vi "ID_ja_aberto.vi"(8 "Conexao nova":refnum<k5>, 9 "Conexao fechada":refnum<k5>, 11 "Entrada Array Conexao":refnum<k5>[](array[refnum])) -> (0 "Saida Array Conexao":refnum<k5>[](array[refnum]))   [LabVIEW 2019]
panel:
  out "iguais":dbl
  # "VI responsável para fazer o controle se o ID recebido é um ID já aberto ou não, e caso ele for fechado, não adicioná-lo"
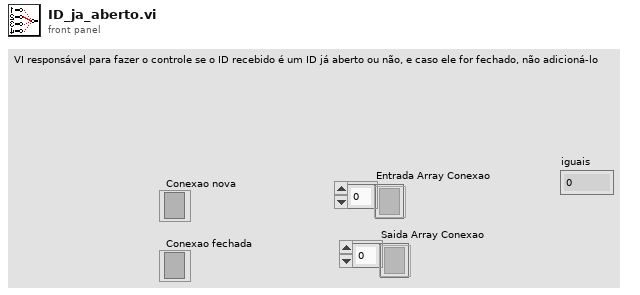
[diagram p1: front panel]
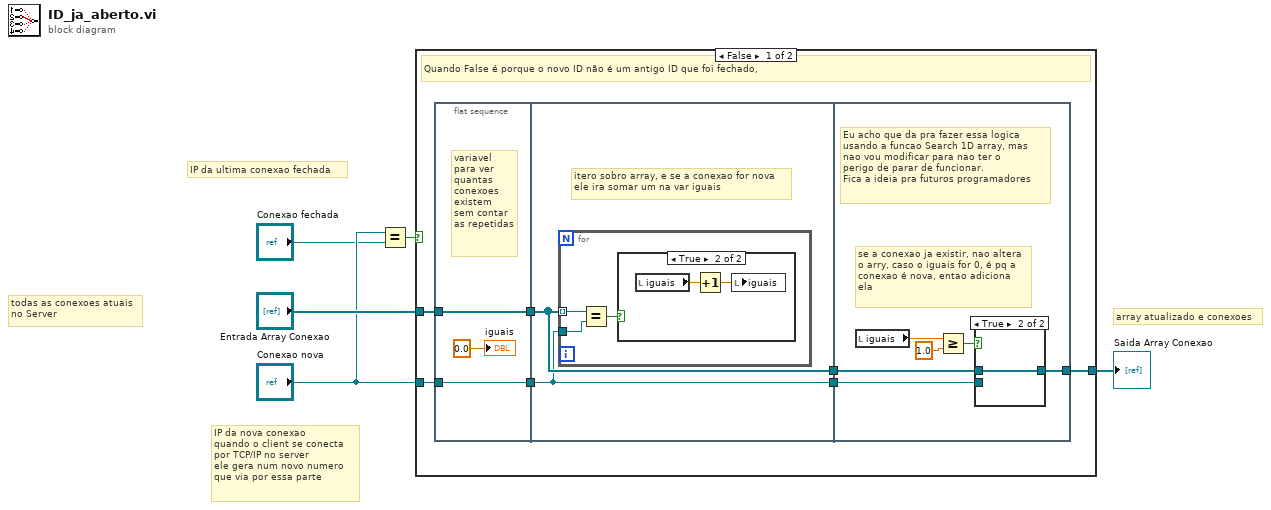
[diagram p0: block diagram]
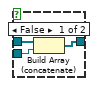
[diagram p3: hidden frame]
diagram:
  # "array atualizado e conexoes"
  # "todas as conexoes atuais\nno Server"
  # "IP da nova conexao\nquando o client se conecta\npor TCP/IP no server\nele gera num novo numero\nque via por essa parte"
  # "IP da ultima conexao fechada"
  n1 = Equal?(x="Conexao nova", y="Conexao fechada") -> (x = y?=w1:bool)
  n2 = case shown="False" w1 {
    tunnel: [w10 w33] -> w5
    tunnel: "Entrada Array Conexao" -> [w8 w33]
    tunnel: "Conexao nova" -> [w6 _]
    frame False {
      # "Quando False é porque o novo ID não é um antigo ID que foi fechado,"
      n3 = flat-sequence {
        tunnel: [w14] -> w9
        tunnel: w8 -> [w14]
        tunnel: [w13] -> w7
        tunnel: w6 -> [w13]
        tunnel: [w17] -> w12
        tunnel: [w16] -> w11
        tunnel: w9 -> [w17]
        tunnel: w7 -> [w16]
        tunnel: w12 -> [w28]
        tunnel: w11 -> [w27]
        tunnel: [w26] -> w10
        frame #0 {
          # "variavel\npara ver\nquantas\nconexoes \nexistem\nsem contar\nas repetidas"
          "iguais" <- 0.0 ("Numeric")
        }
        frame #1 {
          # "itero sobro array, e se a conexao for nova\nele ira somar um na var iguais"
          n4 = for {
            tunnel: w17 -> [w20] mode=indexing
            tunnel: w16 -> [w19]
            n5 = Equal?(x=w20, y=w19) -> (x = y?=w18:bool)
            n6 = case shown="True" w18 {
              frame False {
              }
              frame True {
                n7 = local read "iguais"() -> (w22:dbl)
                n8 = Increment(x=w22) -> (x+1=w21:dbl)
                n9 = local write "iguais"(w21) -> ()
              }
            }
          }
        }
        frame #2 {
          # "Eu acho que da pra fazer essa logica \nusando a funcao Search 1D array, mas \nnao vou modificar para nao ter o\nperigo de parar de funcionar.\nFica a ideia pra futuros programadores"
          # "se a conexao ja existir, nao altera\no arry, caso o iguais for 0, é pq a \nconexao é nova, entao adiciona\nela"
          n10 = local read "iguais"() -> (w25:dbl)
          n11 = Greater Or Equal?(x=w25, y=1.0) -> (x >= y?=w23:bool)
          n12 = case shown="True" w23 {
            tunnel: w28 -> [w31 w32]
            tunnel: w27 -> [w30 _]
            tunnel: [w29 w32] -> w26
            frame False {
              n13 = Build Array (concatenate)(w31, w30) -> (w29:refnum<k5>[])
            }
            frame True {
            }
          }
        }
      }
    }
    frame True {
    }
  }
  "Saida Array Conexao" <- w5
